vi "Route Chassis Clock from Timing Card.vi"(11 "error in":errorcluster) -> (15 "error out":errorcluster)   [LabVIEW 2023, in "RFCalAndFixtureCharact.Common.lvlib"]
uses:
  RFCalAndFixtureCharact.Common.lvlib
  <instrlib>/niSync/niSync.llb/niSync Initialize (Default).vi
  <vilib>/nisyscfg/Close (Filter).vi
  <vilib>/nisyscfg/Close (Resources).vi
  <vilib>/nisyscfg/Close (System).vi
  <vilib>/nisyscfg/nisyscfg.lvlib
  <resource>/objmgr/rfSysapiTags.rc
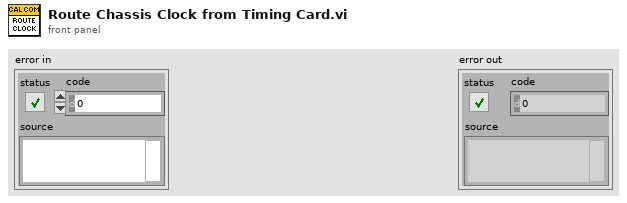
[diagram p1: front panel]
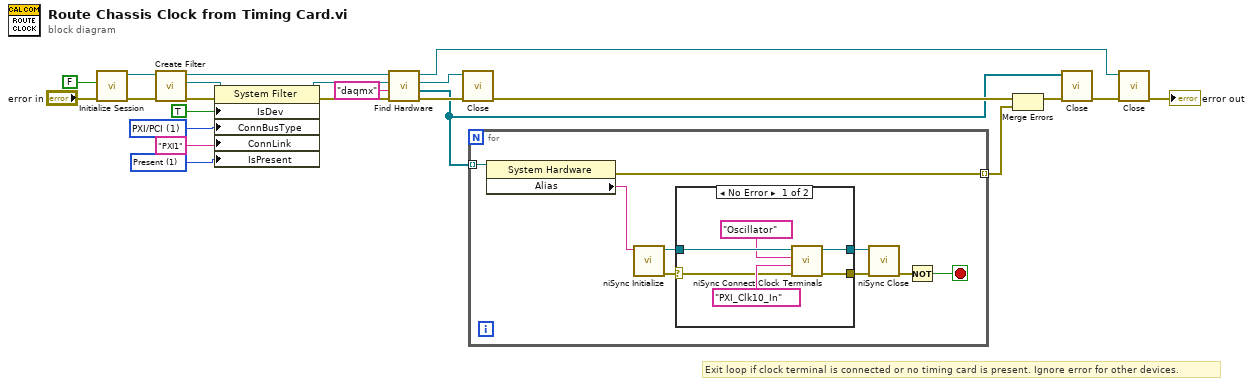
[diagram p0: block diagram]
diagram:
  w2 = 1 items=["Initializing"=-2, "Unknown"=-1, "Not Present"=0, "Present"=1] ("Devices & Chassis:Is Present")
  w12 = u32 1 items=["BuiltIn/System", "PXI/PCI", "USB", "GPIB", "VXI", "Serial", "TCP/IP", "cRIO", "SCXI", "cDAQ", "SwitchBlock", "SCC", "FireWire", "Accessory", "CAN", "SwitchBlock Device"] ("Devices & Chassis:Connects To Bus Type")
  # "Exit loop if clock terminal is connected or no timing card is present. Ignore error for other devices."
  n1 = call <vilib>:"Initialize Session.vi"("error in (no error)"="error in", "Force Property Refresh (T)"=FALSE) -> ("error out"=w19:errorcluster, "Session out"=w17:refnum<k21>)  [unwired: 8 in]
  n2 = call <vilib>:"Create Filter.vi"("error in (no error)"=w19, "Session in"=w17) -> ("error out"=w13:errorcluster, "Filter out"=w14:refnum<k20>, "Session out"=w18:refnum<k21>)  [unwired: 7 in]
  n3 = property class="System Filter"(reference=w14, error in=w13, "IsDev"=TRUE ("Is Chassis"), "ConnBusType"=w12, "ConnLink"="PXI1" ("Chassis"), "IsPresent"=w2) -> (reference out=w16:refnum<k20>, error out=w21:errorcluster)
  n4 = call <vilib>:"Find Hardware.vi"("error in (no error)"=w21, "Experts"="daqmx", "Filter in"=w16, "Session in"=w18) -> ("error out"=w22:errorcluster, "Resources out"=w4:refnum<k20>[], "Filter out"=w20:refnum<k20>, "Session out"=w10:refnum<k21>)  [unwired: 4 in]
  n5 = call-poly <vilib>:"Close.vi"("error in (no error)"=w22, "Filter in"=w20) -> ("error out"=w11:errorcluster)  [unwired: 9 in]
  n6 = for "Map Instrument Name to Intrument Reference" {
    tunnel: w4 -> [w31] mode=indexing
    tunnel: [w32] -> w7 mode=indexing
    stop <- w25 stop-if-true
    n7 = property class="System Hardware"(reference=w31) -> (error out=w32:errorcluster, "Alias"=w27:string)  [unwired: 1 in, 1 out]
    n8 = call-poly <instrlib>:"niSync Initialize.vi"("resource name"=w27) -> ("error out"=w24:errorcluster, "instrument handle out"=w30:refnum<k15>)  [unwired: 9 in]
    n9 = case shown="No Error" w24 {
      selector: w24 -> [w33 w39]
      tunnel: w30 -> [w38 w40]
      tunnel: [w37 w40] -> w29
      tunnel: [w36 w39] -> w28
      frame No Error {
        n10 = call <instrlib>:"niSync Connect Clock Terminals.vi"("error in (no error)"=w33, "destination terminal"="PXI_Clk10_In", "source terminal"="Oscillator", "instrument handle"=w38) -> ("error out"=w36:errorcluster, "instrument handle out"=w37:refnum<k15>)  [unwired: 6 in]
      }
      frame Error {
      }
    }
    n11 = call <instrlib>:"niSync Close.vi"("error in (no error)"=w28, "instrument handle"=w29) -> ("error out"=w26:errorcluster)  [unwired: 9 in]
    n12 = Not(x=w26) -> (.not. x?=w25:bool)
  }
  n13 = Merge Errors(w11, w7) -> (w8:errorcluster)
  n14 = call-poly <vilib>:"Close.vi"("error in (no error)"=w8, "Resources in"=w4) -> ("error out"=w9:errorcluster)  [unwired: 9 in]
  n15 = call-poly <vilib>:"Close.vi"("error in (no error)"=w9, "Session in"=w10) -> ("error out"=→"error out":errorcluster)  [unwired: 9 in]
